vi "UHR-Fleezers Control (host) -Leonardo 04-2018 V1.vi"(0 "Tab Control":T5(tab)=enum."Trap Control (RF)") -> ()   [LabVIEW 2013] (continued)
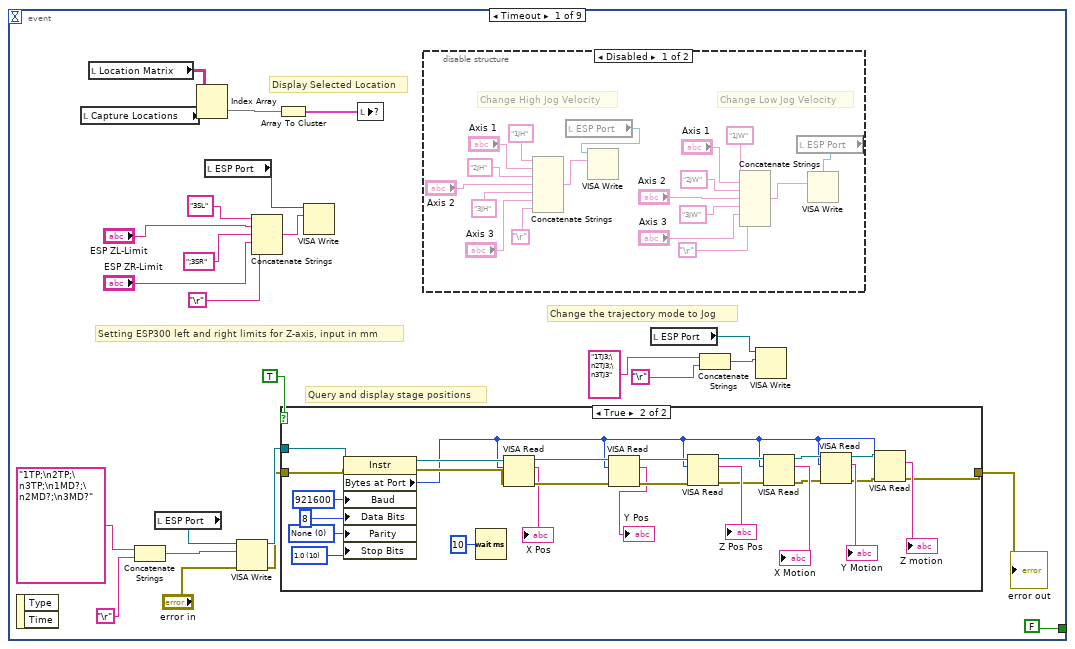
[diagram p2: hidden frame]
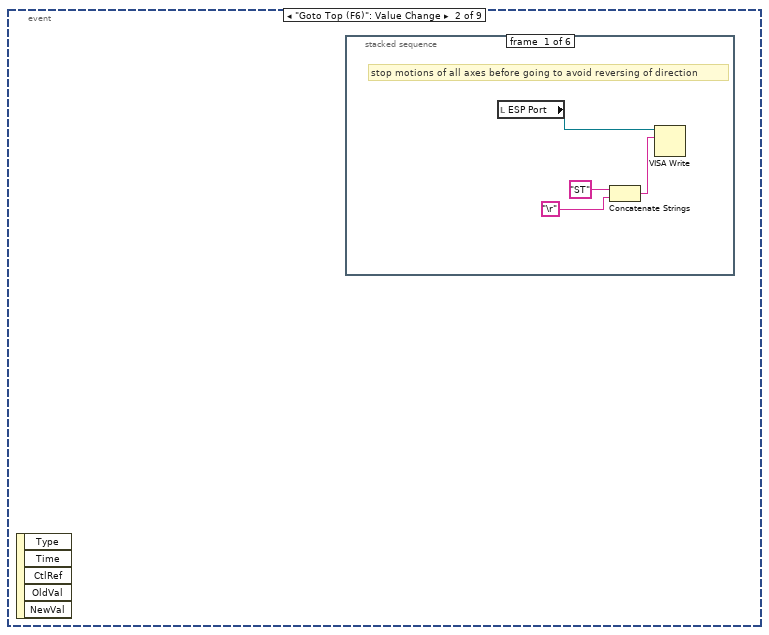
[diagram p5: hidden frame]
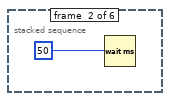
[diagram p6: hidden frame]
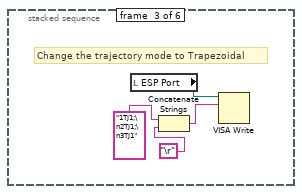
[diagram p7: hidden frame]
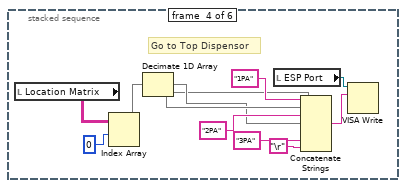
[diagram p8: hidden frame]
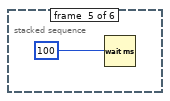
[diagram p9: hidden frame]
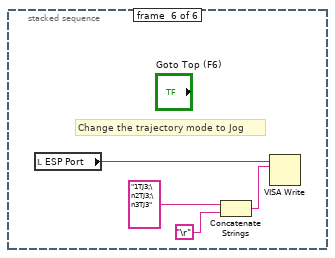
[diagram p10: hidden frame]
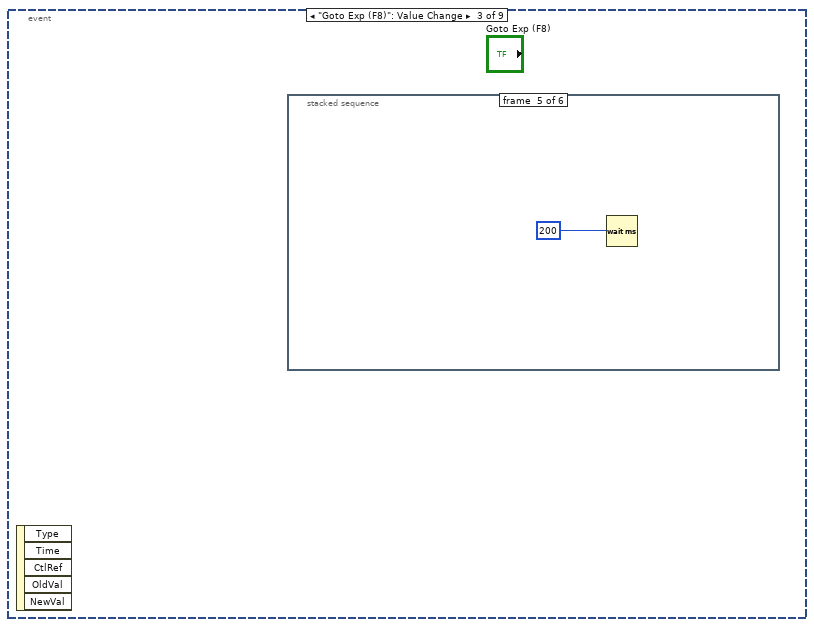
[diagram p11: hidden frame]
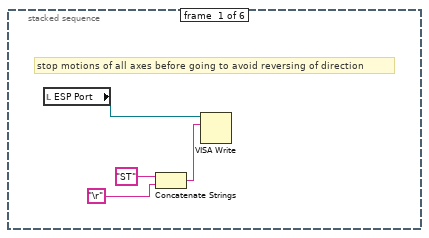
[diagram p12: hidden frame]
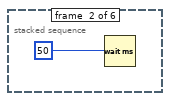
[diagram p13: hidden frame]
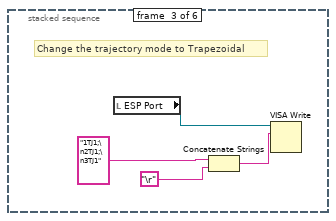
[diagram p14: hidden frame]
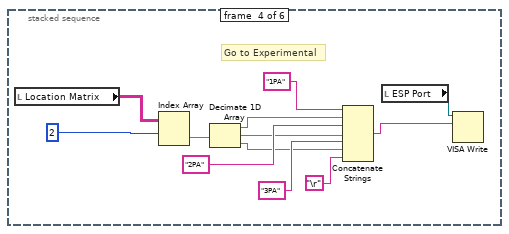
[diagram p15: hidden frame]
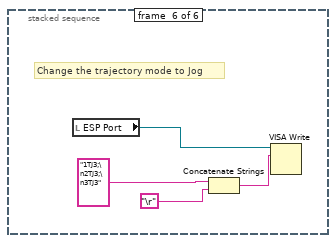
[diagram p16: hidden frame]
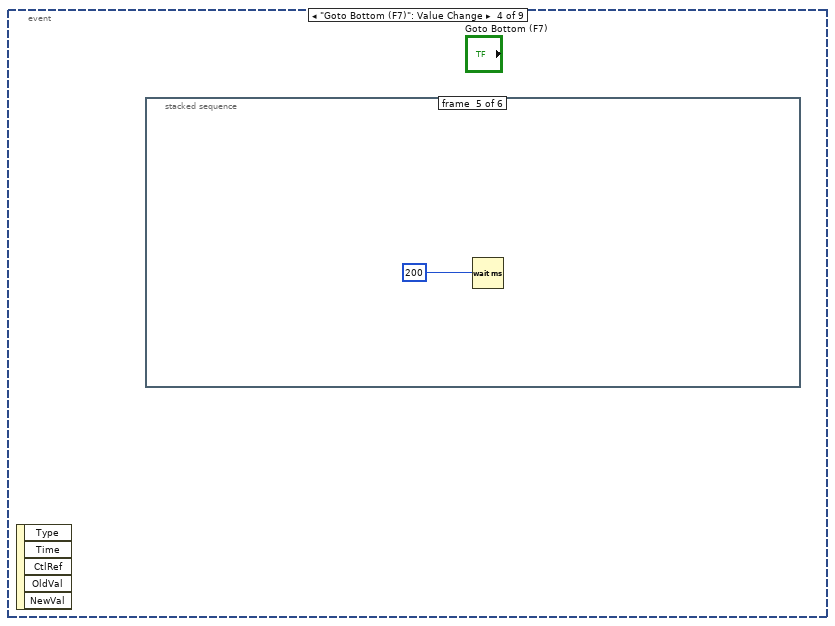
[diagram p17: hidden frame]
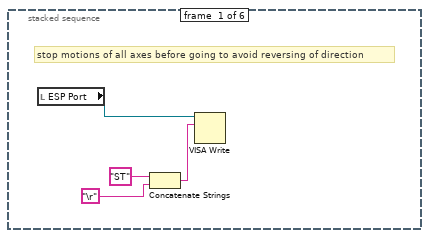
[diagram p18: hidden frame]
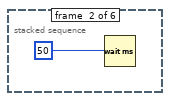
[diagram p19: hidden frame]
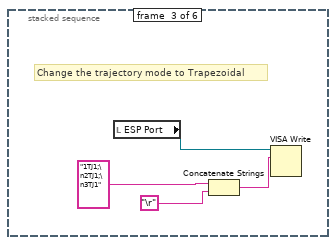
[diagram p20: hidden frame]
                    n2327 = Transpose 2D Array(2D array=w3965) -> (transposed array=w3963:u64[][])
                    n2328 = for {
                      tunnel: w3963 -> [w3968] mode=indexing
                      tunnel: [w3967] -> w3957 mode=indexing
                      tunnel: w3959 -> [w3969]
                      workers-P: _ -> [_]
                      n2329 = call "downsample 1D array - U64.vi"("Ave N"=w3969, "Array In"=w3968) -> ("Array Out"=w3967:u64[])  [unwired: 1 in]
                    }
                    n2330 = Transpose 2D Array(2D array=w3957) -> (transposed array=w3962:u64[][])
                    n2331 = Divide(x=w3960, y=w3959) -> (x/y=w3961:dbl)
                    n2332 = Reshape Array(w3962, w3961) -> (w3958:u64[])
                  }
                }
                n2333 = case shown="True" w3886 {
                  tunnel: w3946 -> [w3978 w3990]
                  tunnel: [w3978 w3982] -> w3942
                  tunnel: "Save ave N" -> [_ w3983]
                  tunnel: w3937 -> [_ w3981]
                  frame False {
                    # "don't downsample data for trap calibration"
                  }
                  frame True {
                    n2334 = Array Size(array=w3990) -> (size(s)=w3984:i32)
                    n2335 = Array Size(array=w3981) -> (size(s)=w3980:i32)
                    n2336 = Divide(x=w3984, y=w3980) -> (x/y=w3988:dbl)
                    n2337 = Reshape Array(w3990, w3988, w3980) -> (w3989:i16[][])
                    n2338 = Transpose 2D Array(2D array=w3989) -> (transposed array=w3987:i16[][])
                    n2339 = for {
                      tunnel: w3987 -> [w3993] mode=indexing
                      tunnel: [w3992] -> w3979 mode=indexing
                      tunnel: w3983 -> [w3991]
                      workers-P: _ -> [_]
                      n2340 = call "downsample 1D array - I16.vi"("Ave N"=w3991, "Array In"=w3993) -> ("Array Out"=w3992:i16[])  [unwired: 1 out]
                    }
                    n2341 = Transpose 2D Array(2D array=w3979) -> (transposed array=w3986:i16[][])
                    n2342 = Divide(x=w3984, y=w3983) -> (x/y=w3985:dbl)
                    n2343 = Reshape Array(w3986, w3985) -> (w3982:i16[])
                  }
                }
                n2344 = Index Array(array=w3908, index=1) -> (element=w3911:waveform(dbl))
                n2345 = Index Array(array=w3908, index=0) -> (element=w3913:waveform(dbl))
                n2346 = Unbundle By Name(w3911) -> ("Y"=w3915:dbl[])
                n2347 = Unbundle By Name(w3913) -> ("Y"=w3923:dbl[])
                n2348 = case "Write trap pos. data" shown="True" w3889 {
                  tunnel: w3888 -> [_ w3971]
                  tunnel: w3884 -> [_ w3970]
                  frame False {
                  }
                  frame True {
                    n2349 = Write to Binary File(file (use dialog)=w3971, data=w3970, 5:FALSE ("prepend array or string size? (T)"), 9:T30."big-endian, network order" ("byte order (0:big-endian, network order)")) -> ()  [unwired: 1 in, 4 out]
                  }
                }
                n2350 = Write to Binary File(file (use dialog)=w3949, data=w3942, 5:FALSE ("prepend array or string size? (T)"), 9:T30."big-endian, network order" ("byte order (0:big-endian, network order)")) -> ()  [unwired: 1 in, 4 out]
                n2351 = feedback #26(w3915) -> (w3917:dbl[])
                n2352 = Build Array (concatenate)(w3917, w3915) -> (w3916:dbl[])
                n2353 = Select(t=w3915, s=w3891, f=w3916) -> (s? t:f=w3901:dbl[])
                n2354 = feedback-in #26(w3901) -> ()
                n2355 = feedback #27(w3923) -> (w3936:dbl[])
                n2356 = Build Array (concatenate)(w3936, w3923) -> (w3935:dbl[])
                n2357 = Select(t=w3923, s=w3891, f=w3935) -> (s? t:f=w3910:dbl[])
                n2358 = feedback-in #27(w3910) -> ()
                n2359 = Divide(x=w3950, y=w3951) -> (x/y=w3953:dbl)
                n2360 = Multiply(x=w3953, y=100.0) -> (x*y=w3952:dbl)
                n2361 = Build Array(w3910, w3901) -> (→"Saved APD":dbl[][])
                n2362 = Array Size(array=w3910) -> (size(s)=w3928:i32)
                n2363 = Unbundle By Name(w3930) -> ("Y"=w3934:dbl[])
                n2364 = Subtract(x=w3928, y="N pts to average") -> (x-y=w3904:i32)
                n2365 = Multiply(x="N pts to average", y=u16 2) -> (x*y=w3905:u16)
                n2366 = Subtract(x=w3928, y=w3905) -> (x-y=w3903:i32)
                n2367 = feedback #28(w3934) -> (w3933:dbl[])
                n2368 = Build Array (concatenate)(w3933, w3934) -> (w3932:dbl[])
                n2369 = Select(t=w3934, s=w3891, f=w3932) -> (s? t:f=w3931:dbl[])
                "Trap Delta Graph" <- w3931
                n2370 = feedback-in #28(w3931) -> ()
                n2371 = Array Subset(array=w3910, index=w3904, length="N pts to average") -> (w3927:dbl[])
                n2372 = Array Subset(array=w3910, index=w3903, length="N pts to average") -> (w3926:dbl[])
                n2373 = Array Subset(array=w3901, index=w3904, length="N pts to average") -> (w3907:dbl[])
                n2374 = Array Subset(array=w3901, index=w3903, length="N pts to average") -> (w3906:dbl[])
                n2375 = call-poly <vilib>:"Mean.vi"("X"=w3927) -> ("mean"=w3925:dbl)  [unwired: 1 out]
                n2376 = call-poly <vilib>:"Mean.vi"("X"=w3907) -> ("mean"=w3900:dbl)  [unwired: 1 out]
                n2377 = call-poly <vilib>:"Mean.vi"("X"=w3926) -> ("mean"=w3924:dbl)  [unwired: 1 out]
                n2378 = call-poly <vilib>:"Mean.vi"("X"=w3906) -> ("mean"=w3899:dbl)  [unwired: 1 out]
                n2379 = Subtract(x=w3900, y=w3899) -> (x-y=w3890:dbl)
                "Delta Fl. 2" <- w3890
                n2380 = Subtract(x=w3925, y=w3924) -> (x-y=w3922:dbl)
                "Delta Fl. 1" <- w3922
                n2381 = Initialize Array(w3922, 1 ("dimension size")) -> (w3919:dbl[])
                n2382 = Initialize Array(w3890, 1 ("dimension size")) -> (w3896:dbl[])
                n2383 = feedback #29(w3919) -> (w3920:dbl[])
                n2384 = Build Array (concatenate)(w3920, w3919) -> (w3918:dbl[])
                n2385 = feedback #30(w3896) -> (w3897:dbl[])
                n2386 = Build Array (concatenate)(w3897, w3896) -> (w3895:dbl[])
                n2387 = Select(t=w3919, s=w3891, f=w3918) -> (s? t:f=w3894:dbl[])
                n2388 = feedback-in #29(w3894) -> ()
                n2389 = Select(t=w3896, s=w3891, f=w3895) -> (s? t:f=w3893:dbl[])
                n2390 = feedback-in #30(w3893) -> ()
                n2391 = Build Array(w3894, w3893) -> (→"Save APD Deriv":dbl[][])
              }
            }
            "Progress" <- w3867
            "Progress 2" <- w3867
          }
        }
      }
    }
    n2392 = Divide(x=w2248, y=w2249) -> (x/y=w2239:ext)
    "Trap 2 amplitude" <- w2239
    n2393 = Bundle By Name(cluster=w2502, "Green FB Ch 0"=w2501, "Green FB Ch 1"=w2500) -> (w2486:T49)
    "Green FB Signals (V)" <- w2486
    n2394 = case shown="True" w2241 {
      tunnel: w2240 -> [_ w2591]
      tunnel: w2239 -> [_ w2590]
      frame False {
      }
      frame True {
        w2592 = 50.0
        n2395 = Greater?(x=w2590, y=w2592) -> (0:w2588:bool)
        n2396 = Greater?(x=w2591, y=w2592) -> (0:w2589:bool)
        n2397 = Or(x=w2589, y=w2588) -> (x .or. y?=w2587:bool)
        n2398 = case shown="True" w2587 {
          frame False {
          }
          frame True {
            n2399 = property on="All FB On/Off" class="Bool (strict)"("Val(Sgnl)"=FALSE) -> ()  [unwired: 2 in, 2 out]
            "Feedback overload" <- TRUE
          }
        }
      }
    }
    n2400 = Unbundle By Name(w2486) -> ("Green FB Ch 2"=→"Green FB Plot":dbl)
    n2401 = local read "wait to reset values"() -> (w2570:bool)
    n2402 = Not(x=w2567) -> (.not. x?=w2571:bool)
    n2403 = And(x=w2571, y=w2570) -> (x .and. y?=w2572:bool)
    n2404 = case "Part of MCL raster scanning: returns to initial positions after scan done" shown="True" w2572 {
      tunnel: w2575 -> [w3416 w3423]
      tunnel: [w3416 w3422] -> w2574
      tunnel: w2569 -> [w3415 w3421]
      tunnel: [w3415 w3420] -> w2568
      frame False {
      }
      frame True {
        w3431 = 10.0 ("y")
        w3430 = 32767.0 ("y")
        # "to return scan values\nafter a synchronous \nAOM scan"
        n2405 = local read "AO2"() -> (w3424:dbl)
        n2406 = local read "AO1"() -> (w3425:dbl)
        n2407 = local write "wait to reset values"(FALSE ("wait to reset values")) -> ()
        n2408 = Multiply(x=w3425, y=w3430) -> (x*y=w3427:dbl)
        n2409 = Multiply(x=w3424, y=w3430) -> (x*y=w3429:dbl)
        n2410 = Divide(x=w3427, y=w3431) -> (x/y=w3426:dbl)
        n2411 = Divide(x=w3429, y=w3431) -> (x/y=w3428:dbl)
        n2412 = To Word Integer(number=w3426) -> (16bit integer=w3432:i16)
        n2413 = To Word Integer(number=w3428) -> (16bit integer=w3433:i16)
        n2414 = local read "Total Counts (ticks)"() -> (w3417:u32)
        n2415 = xnode "Read/Write Control"("FPGA VI Reference In"=w3423, "error in"=w3421, "AO1 (Y)"=w3432, "AO2 (X)"=w3433, "MCL count"=w3417) -> ("FPGA VI Reference Out"=w3422:T20, "error out"=w3420:errorcluster)
        n2416 = local read "Scan Range (V)\n(of steps)"() -> (w3418:dbl)
        n2417 = property on="Scan Range (V)\n(of steps)" class="DigNum (strict)"("Val(Sgnl)"=w3418) -> ()  [unwired: 2 in, 2 out]
      }
    }
    n2418 = node-c288() -> ()  [unwired: 2 out]
  }
  n2419 = node-c288(3 ("Processor")) -> (w107:T25)  [unwired: 3 out]
  n2420 = timed-loop "Oscillate AOD (debugging)" {
    tunnel: w59 -> [w3995]
    tunnel: [w3994] -> w71
    timing: w107 -> [_]
    timing-out: [_] -> w106
    stop <- w3994 stop-if-true
    n2421 = node-c288() -> ()  [unwired: 2 out]
    n2422 = event shown="[0] \"Oscillate Set 2\", \"Fish for Tether\": Value Change" {
      selector: _ -> [_ _ _]
      dyn-events: _ -> [_ _ _]
      timeout: _ -> [_ _ _]
      tunnel: w3995 -> [w4002 _ _]
      tunnel: [FALSE ("Stop All") _ w4270] -> w3994
      event "Oscillate Set 2", "Fish for Tether": Value Change {
        n2423 = event-data() -> ()  [unwired: 6 out]
        n2424 = local read "Oscillate Set 2"() -> (w4001:bool)
        n2425 = Or(x=w4001, y="Fish for Tether") -> (x .or. y?=w3999:bool)
        n2426 = case shown="True" w3999 {
          tunnel: w4002 -> [_ w4005]
          tunnel: "Fish for Tether" -> [_ w4004]
          frame False {
          }
          frame True {
            n2427 = case shown="True" w4004 {
              frame False {
              }
              frame True {
                n2428 = local write "Scan axis 2"(TRUE) -> ()
                n2429 = local write "Tether"(FALSE ("Tether")) -> ()
              }
            }
            n2430 = node-c288("Period") -> (w4007:T25)  [unwired: 3 out]
            n2431 = timed-loop "Oscillate AOD" {
              timing: w4007 -> [_]
              timing-out: [_] -> w4006
              tunnel: w4005 -> [w4017]
              tunnel: w4004 -> [w4016]
              i -> [w4019]
              stop <- w4015 stop-if-true
              n2432 = node-c288() -> (w4018:i64)  [unwired: 1 out]
              n2433 = flat-sequence {
                tunnel: w4019 -> [w4045]
                tunnel: w4018 -> [w4044]
                tunnel: w4017 -> [w4028]
                tunnel: w4016 -> [w4030]
                tunnel: [w4030] -> w4014
                tunnel: [w4029] -> w4013
                tunnel: [w4027] -> w4012
                tunnel: [w4024] -> w4010
                tunnel: w4014 -> [w4081]
                tunnel: w4013 -> [w4079]
                tunnel: w4012 -> [w4078]
                tunnel: [w4077] -> w4011
                tunnel: w4010 -> [w4076]
                tunnel: [w4145] -> w4015
                tunnel: w4011 -> [w4143]
                frame #0 {
                  n2434 = Divide(x=w4044, y=i64 1000) -> (x/y=w4039:dbl)
                  n2435 = Multiply(x=w4039, y=w4045) -> (x*y=w4041:dbl)
                  n2436 = Multiply(x="Osc. freq. (Hz)", y=6.283185307179586) -> (x*y=w4042:dbl)
                  n2437 = Multiply(x=w4042, y=w4041) -> (x*y=w4026:dbl)
                  n2438 = local read "BD 1 Frequency 2 (MHz)"() -> (w4023:dbl)
                  n2439 = local read "BD 1 Frequency 1 (MHz)"() -> (w4020:dbl)
                  n2440 = case shown="True" w4030 {
                    tunnel: w4026 -> [w4051 w4058]
                    tunnel: w4023 -> [_ w4068]
                    tunnel: [w4048 w4052] -> w4031
                    tunnel: [FALSE w4061] -> w4027
                    tunnel: [0.0 w4054] -> w4024
                    tunnel: w4020 -> [_ w4053]
                    frame False {
                      n2441 = Sine(x=w4051) -> (sin(x)=w4049:dbl)
                      n2442 = Multiply(x=w4049, y="Osc. amp. (MHz)") -> (x*y=w4048:dbl)
                    }
                    frame True {
                      n2443 = Cosine(x=w4058) -> (cos(x)=w4071:dbl)
                      n2444 = Subtract(x=w4068, y=w4053) -> (x-y=w4067:dbl)
                      n2445 = Decrement(x=w4071) -> (x-1=w4070:dbl)
                      n2446 = Subtract(x=w4067, y="Closest Delta (MHz)") -> (x-y=w4064:dbl)
                      n2447 = Divide(x=w4070, y=2.0) -> (x/y=w4065:dbl)
                      n2448 = Multiply(x=w4065, y=w4064) -> (x*y=w4052:dbl)
                      n2449 = local read "Vec Mean of T1 T2"() -> (w4060:dbl[])
                      n2450 = Greater?(x=w4060, y="Stop F (pN)") -> (0:w4062:bool[])
                      n2451 = Or Array Elements(Boolean array=w4062) -> (logical OR=w4061:bool)
                      n2452 = Divide(x=w4058, y=6.283185307179586) -> (x/y=w4057:dbl)
                      n2453 = Round Toward +Infinity(x=w4057) -> (ceil(x): smallest int >= x=w4054:dbl)
                      "Attempts" <- w4054
                      n2454 = Greater?(x=w4054, y="Attempt Limit") -> (0:w4056:bool)
                      n2455 = case shown="True" w4056 {
                        frame False {
                        }
                        frame True {
                          n2456 = local write "Fish for Tether"(FALSE ("Fish for Tether")) -> ()
                          n2457 = call <vilib>:"Beep.vi"() -> ()  [unwired: 3 in, 9 out]
                          n2458 = local read "Messages"() -> (w4073:string)
                          n2459 = call "Update messages.vi"("Message to add"="Tether fishing timeout." ("Messages"), "Old message string"=w4073) -> ("New message string"=→"Messages":string)
                        }
                      }
                    }
                  }
                  n2460 = local read "Y RF Frequency Limits (MHz)"() -> (w4032:T16)
                  n2461 = local read "X RF Frequency Limits (MHz)"() -> (w4033:T16)
                  n2462 = local read "BD 1 Frequency 3 (MHz)"() -> (w4038:dbl)
                  n2463 = local read "BD 2 Frequency 2 (MHz)"() -> (w4022:dbl)
                  n2464 = Select(t=w4023, s="Scan axis 2", f=w4022) -> (s? t:f=w4034:dbl)
                  n2465 = Add(x=w4031, y=w4034) -> (x+y=w4029:dbl)
                  n2466 = Select(t=w4029, s="Scan axis 2", f=w4023) -> (s? t:f=w4021:dbl)
                  n2467 = Select(t=w4022, s="Scan axis 2", f=w4029) -> (s? t:f=w4036:dbl)
                  n2468 = local read "BD 2 Frequency 3 (MHz)"() -> (w4037:dbl)
                  n2469 = call "set RF board frequency - interlace.vi"("Board 2 Frequency Limits"=w4032, "Board 1 Frequency Limits"=w4033, "FPGA VI Reference In"=w4028, "Board 2 Frequency 3 (MHz)"=w4037, "Board 1 Frequency 3 (MHz)"=w4038, "Board 2 Frequency 2 (MHz)"=w4022, "Board 2 Frequency 1 (MHz)"=w4036, "Board 1 Frequency 2 (MHz)"=w4021, "Board 1 Frequency 1  (MHz)"=w4020) -> ()  [unwired: 1 in, 2 out]
                }
                frame #1 {
                  n2470 = And(x=w4081, y=w4078) -> (x .and. y?=w4080:bool)
                  n2471 = case "Only if were fishing and now formed tether" shown="True" w4080 {
                    tunnel: w4079 -> [w4083 w4095]
                    tunnel: [w4082 w4094] -> w4077
                    tunnel: w4076 -> [_ w4090]
                    frame False {
                      n2472 = local read "Fish for Tether"() -> (w4082:bool)
                      n2473 = case shown="True" w4082 {
                        tunnel: w4083 -> [_ _]
                        frame False {
                        }
                        frame True {
                        }
                      }
                    }
                    frame True {
                      w4094 = FALSE ("Fish for Tether")
                      n2474 = call <vilib>:"Beep.vi"() -> ()  [unwired: 3 in, 9 out]
                      n2475 = Number To Decimal String(number=w4090, width (-)=i16 1) -> (decimal integer string=w4088:string)
                      n2476 = case shown="\"2\", \"3\", \"4\", \"5\", \"6\"" "Then..." {
                        selector: "Then..." -> [_ w4098]
                        tunnel: w4095 -> [w4097 _]
                        frame "1", Default {
                          # "do nothing"
                          n2477 = property on="BD 1 Frequency 1 (MHz)" class="DigNum (strict)"("Val(Sgnl)"=w4097) -> ()  [unwired: 2 in, 2 out]
                        }
                        frame "2", "3", "4", "5", "6" {
                          n2478 = flat-sequence {
                            tunnel: w4098 -> [w4100]
                            frame #0 {
                              n2479 = property on="Trap Delta (MHz)" class="DigNum (strict)"("Val(Sgnl)"="Move to Delta 1 (MHz)") -> ()  [unwired: 2 in, 2 out]
                            }
                            frame #1 {
                              n2480 = case shown="\"5\", \"6\"" w4100 {
                                selector: w4100 -> [w4103 w4113 _]
                                frame "3", "4" {
                                n2481 = flat-sequence {
                                tunnel: w4103 -> [w4104]
                                tunnel: [w4104] -> w4101
                                tunnel: [w4106] -> w4102
                                tunnel: w4101 -> [w4106]
                                tunnel: w4102 -> [w4110]
                                frame #0 {
                                n2482 = property on="Green Laser ON/Interlacing" class="Bool (strict)"("Val(Sgnl)"=TRUE ("Value (Signaling)")) -> ()  [unwired: 2 in, 2 out]
                                }
                                frame #1 {
                                n2483 = Multiply(x="Wait Before Save (s)", y=u32 1000 ("x")) -> (x*y=w4108:u32)
                                n2484 = Wait (ms)(milliseconds to wait=w4108) -> ()  [unwired: 1 out]
                                }
                                frame #2 {
                                n2485 = property on="Start Saving" class="Bool (strict)"("Value"=TRUE ("Start Saving")) -> ()  [unwired: 2 in, 2 out]
                                n2486 = case shown="Default" w4110 {
                                frame Default {
                                }
                                frame "4" {
                                n2487 = property on="Fl. Triggered..." class="Bool (strict)"("Val(Sgnl)"=TRUE ("Value (Signaling)")) -> ()  [unwired: 2 in, 2 out]
                                }
                                }
                                }
                                }
                                }
                                frame "5", "6" {
                                n2488 = stacked-sequence {
                                tunnel: w4113 -> [_ _ _ _ _ _ _ _ w4130 _ _]
                                frame #0 {
                                n2489 = Replace Array Subset(array=u32[] [0] ("Index Values"), new element="Raster Set Upon Tether", index=0) -> (w4114:u32[])
                                n2490 = property on="Saved AOD Raster Scan Parameter Sets" class="Arr (strict)"("Index Values"=w4114) -> ()  [unwired: 2 in, 2 out]
                                }
                                frame #1 {
                                n2491 = Wait (ms)(milliseconds to wait=u32 500) -> ()  [unwired: 1 out]
                                }
                                frame #2 {
                                n2492 = property on="Load parameters" class="Bool (strict)"("Val(Sgnl)"=TRUE ("Value (Signaling)")) -> ()  [unwired: 2 in, 2 out]
                                }
                                frame #3 {
                                n2493 = Wait (ms)(milliseconds to wait=u32 500) -> ()  [unwired: 1 out]
                                }
                                frame #4 {
                                n2494 = property on="Trap Raster Scan" class="Bool (strict)"("Val(Sgnl)"=TRUE ("Value (Signaling)")) -> ()  [unwired: 2 in, 2 out]
                                }
                                frame #5 {
                                n2495 = Wait (ms)(milliseconds to wait=u32 2000) -> ()  [unwired: 1 out]
                                }
                                frame #6 {
                                n2496 = while {
                                stop <- w4125 stop-if-true
                                n2497 = local read "Raster Scanning..."() -> (w4124:bool)
                                n2498 = local read "Saving..."() -> (w4127:bool)
                                n2499 = Wait (ms)(milliseconds to wait=u32 100) -> ()  [unwired: 1 out]
                                n2500 = Not(x=w4127) -> (.not. x?=w4126:bool)
                                n2501 = Not(x=w4124) -> (.not. x?=w4123:bool)
                                n2502 = And(x=w4126, y=w4123) -> (x .and. y?=w4125:bool)
                                }
                                }
                                frame #7 {
                                n2503 = property on="Trap Delta (MHz)" class="DigNum (strict)"("Val(Sgnl)"="Move to Delta 2 (MHz)") -> ()  [unwired: 2 in, 2 out]
                                }
                                frame #8 {
                                n2504 = local read "Tether"() -> (w4131:bool)
                                n2505 = case shown="True" w4131 {
                                tunnel: w4130 -> [_ w4132]
                                frame False {
                                }
                                frame True {
                                n2506 = flat-sequence {
                                tunnel: w4132 -> [w4134]
                                frame #0 {
                                n2507 = Wait (ms)(milliseconds to wait=u32 500) -> ()  [unwired: 1 out]
                                }
                                frame #1 {
                                n2508 = case shown="\"6\"" w4134 {
                                frame Default {
                                }
                                frame "6" {
                                n2509 = property on="Green Laser ON/Interlacing" class="Bool (strict)"("Val(Sgnl)"=TRUE ("Green Laser ON/Interlacing")) -> ()  [unwired: 2 in, 2 out]
                                }
                                }
                                }
                                frame #2 {
                                n2510 = Wait (ms)(milliseconds to wait=u32 500) -> ()  [unwired: 1 out]
                                }
                                frame #3 {
                                n2511 = local write "Start Saving"("Save at end (5, 6)") -> ()
                                }
                                }
                                }
                                }
                                }
                                frame #9 {
                                n2512 = local read "Bead Sep. Int. Time (s)"() -> (w4140:dbl)
                                n2513 = Multiply(x=w4140, y=1000.0) -> (x*y=w4139:dbl)
                                n2514 = Wait (ms)(milliseconds to wait=w4139) -> ()  [unwired: 1 out]
                                }
                                frame #10 {
                                n2515 = property on="Rescale on Mean" class="Bool (strict)"("Val(Sgnl)"=TRUE ("Value (Signaling)")) -> ()  [unwired: 2 in, 2 out]
                                }
                                }
                                }
                                frame "2", Default {
                                }
                              }
                            }
                          }
                        }
                      }
                      n2516 = Concatenate Strings("Formed tether in ", w4088, " attempt(s)." ("string")) -> (w4085:string)
                      n2517 = local read "Messages"() -> (w4092:string)
                      n2518 = local write "Fish for Tether"(w4094) -> ()
                      n2519 = call "Update messages.vi"("Message to add"=w4085, "Old message string"=w4092) -> ("New message string"=w4091:string)
                      n2520 = local write "Messages"(w4091) -> ()
                      n2521 = Get Date/Time In Seconds() -> (seconds since 1Jan1904=→"Time tether formed":timestamp)
                      "Tether" <- "Tether Alarm?"
                    }
                  }
                }
                frame #2 {
                  n2522 = local read "Oscillate Set 2"() -> (w4144:bool)
                  n2523 = local read "Stop All"() -> (w4146:bool)
                  n2524 = Not Or(1:w4143, 2:w4144) -> (0:w4142:bool)
                  n2525 = Compound Arithmetic op=OR(w4146, w4142) -> (w4145:bool)
                }
              }
              n2526 = node-c288() -> ()  [unwired: 2 out]
            }
            n2527 = node-c288(w4006) -> ()  [unwired: 1 out]
          }
        }
      }
      event "Fl. Triggered...": Value Change {
        n2528 = event-data() -> ()  [unwired: 7 out]
        n2529 = case shown="True" "Fl. Triggered..." {
          frame False {
          }
          frame True {
            n2530 = node-c288() -> (w4158:T25)  [unwired: 4 out]
            n2531 = timed-loop {
              timing: w4158 -> [_]
              timing-out: [_] -> w4157
              tunnel: "Action" -> [w4162]
              shift-right: [w4159] -> _
              shift-left: u8 255 -> [w4161]
              stop <- w4163 stop-if-true
              n2532 = node-c288() -> ()  [unwired: 2 out]
              n2533 = flat-sequence {
                tunnel: w4162 -> [w4175]
                tunnel: w4161 -> [w4172]
                tunnel: [w4171] -> w4160
                tunnel: [w4261] -> w4163
                tunnel: w4160 -> [w4260]
                tunnel: [w4260] -> w4159
                frame #0 {
                  n2534 = local read "Delta Fl. 2"() -> (w4166:dbl)
                  n2535 = local read "Delta Fl. 1"() -> (w4167:dbl)
                  n2536 = Select(t=w4167, s="APD to Watch", f=w4166) -> (s? t:f=w4165:dbl)
                  n2537 = Multiply(x="Fl. Delta Thresh. (kHz)", y=1000.0) -> (x*y=w4174:dbl)
                  n2538 = Greater?(x=w4165, y=w4174) -> (0:w4169:bool)
                  n2539 = Or(x="Force Yank", y=w4169) -> (x .or. y?=w4170:bool)
                  n2540 = case shown="True" w4170 {
                    tunnel: w4175 -> [_ w4185]
                    tunnel: w4172 -> [w4177 w4181]
                    tunnel: [w4177 w4178] -> w4171
                    frame False {
                    }
                    frame True {
                      n2541 = flat-sequence {
                        tunnel: w4182 -> [w4191]
                        tunnel: [w4191] -> w4186
                        tunnel: w4185 -> [w4190]
                        tunnel: [w4190] -> w4184
                        tunnel: [w4189] -> w4183
                        tunnel: w4181 -> [w4188]
                        tunnel: [w4187] -> w4180
                        tunnel: w4186 -> [w4216]
                        tunnel: w4184 -> [w4215]
                        tunnel: w4183 -> [w4214]
                        tunnel: w4180 -> [w4213]
                        tunnel: [w4213] -> w4179
                        tunnel: w4179 -> [w4258]
                        tunnel: [w4258] -> w4178
                        frame #0 {
                          n2542 = call <vilib>:"Beep.vi"() -> ()  [unwired: 3 in, 9 out]
                          n2543 = local write "Waiting"(FALSE ("Waiting")) -> ()
                          n2544 = Increment(x=w4188) -> (x+1=w4187:u8)
                          n2545 = case shown="\"Yank\"" w4190 {
                            tunnel: w4187 -> [_ _ w4197]
                            frame "Image" {
                              n2546 = property on="Confocal Image" class="Bool (strict)"("Val(Sgnl)"=TRUE ("Value (Signaling)")) -> ()  [unwired: 2 in, 2 out]
                            }
                            frame "Alarm", Default {
                            }
                            frame "Yank" {
                              n2547 = flat-sequence {
                                tunnel: w4197 -> [w4200]
                                tunnel: [w4199] -> w4196
                                tunnel: ["N Array El"] -> w4195
                                tunnel: w4196 -> [w4210]
                                tunnel: w4195 -> [w4206]
                                frame #0 {
                                n2548 = Multiply(x="Yank Delay (s)", y=1000.0) -> (x*y=w4203:dbl)
                                n2549 = Quotient & Remainder(x=w4200, y="N Array El") -> (x-y*floor(x/y)=w4199:u8)  [unwired: 1 out]
                                n2550 = Wait (ms)(milliseconds to wait=w4203) -> ()  [unwired: 1 out]
                                }
                                frame #1 {
                                n2551 = Random Number (0-1)() -> (number: 0 to 1=w4207:dbl)
                                n2552 = Multiply(x=w4206, y=w4207) -> (x*y=w4205:dbl)
                                n2553 = Round Toward -Infinity(1:w4205) -> (0:w4204:dbl)
                                n2554 = Select(t=w4204, s="Random Choice", f=w4210) -> (s? t:f=w4208:dbl)
                                n2555 = Index Array(array="Yank to Delta Array (MHz)", index=w4208) -> (element=w4211:dbl)
                                n2556 = property on="Trap Delta (MHz)" class="DigNum (strict)"("Val(Sgnl)"=w4211) -> ()  [unwired: 2 in, 2 out]
                                }
                              }
                            }
                          }
                          n2557 = local read "Time (s)"() -> (w4189:dbl)
                          "Fl. High" <- TRUE ("Yanking")
                        }
                        frame #1 {
                          n2558 = node-c288() -> (w4218:T25)  [unwired: 4 out]
                          n2559 = timed-loop {
                            timing: w4218 -> [_]
                            timing-out: [_] -> w4217
                            tunnel: w4216 -> [w4234]
                            tunnel: w4215 -> [w4232]
                            tunnel: w4214 -> [w4231]
                            stop <- w4233 stop-if-true
                            n2560 = node-c288() -> ()  [unwired: 2 out]
                            n2561 = local read "Fl. Delta Thresh. (kHz)"() -> (w4226:dbl)
                            n2562 = local read "Fl. Triggered..."() -> (w4235:bool)
                            n2563 = local read "Delta Fl. 1"() -> (w4222:dbl)
                            n2564 = local read "Delta Fl. 2"() -> (w4220:dbl)
                            n2565 = local read "Stop All"() -> (w4229:bool)
                            n2566 = local read "APD to Watch"() -> (w4221:bool)
                            n2567 = Select(t=w4222, s=w4221, f=w4220) -> (s? t:f=w4219:dbl)
                            n2568 = Not(x=w4235) -> (.not. x?=w4230:bool)
                            n2569 = Multiply(x=w4226, y=1000.0) -> (x*y=w4225:dbl)
                            n2570 = Negate(x=w4225) -> (-x=w4224:dbl)
                            n2571 = Less?(x=w4219, y=w4224) -> (x < y?=w4228:bool)
                            n2572 = Compound Arithmetic op=OR(w4228, w4229, w4230, "Force Reset") -> (w4233:bool)
                            n2573 = case shown="True" w4233 {
                              tunnel: w4234 -> [_ w4246]
                              tunnel: w4232 -> [_ w4245]
                              tunnel: w4231 -> [_ w4243]
                              frame False {
                              }
                              frame True {
                                n2574 = case shown="\"Yank\"" w4245 {
                                tunnel: w4246 -> [_ w4247]
                                frame "Image", Default {
                                }
                                frame "Yank" {
                                n2575 = flat-sequence {
                                tunnel: [w4252] -> w4248
                                tunnel: w4247 -> [w4252]
                                tunnel: w4248 -> [w4253]
                                frame #0 {
                                n2576 = local read "Yank Delay (s)"() -> (w4251:dbl)
                                n2577 = Multiply(x=w4251, y=1000.0) -> (x*y=w4249:dbl)
                                n2578 = Wait (ms)(milliseconds to wait=w4249) -> ()  [unwired: 1 out]
                                }
                                frame #1 {
                                n2579 = property on="Trap Delta (MHz)" class="DigNum (strict)"("Val(Sgnl)"=w4253) -> ()  [unwired: 2 in, 2 out]
                                }
                                }
                                }
                                }
                                n2580 = local read "Time (s)"() -> (w4244:dbl)
                                n2581 = Subtract(x=w4244, y=w4243) -> (x-y=w4240:dbl)
                                "Duration (s)" <- w4240
                                n2582 = Number To Decimal String(number=w4240, width (-)=i16 0) -> (decimal integer string=w4238:string)
                                n2583 = Concatenate Strings(w4238, " s fluorescence event." ("string")) -> (w4236:string)
                                n2584 = local read "Messages"() -> (w4242:string)
                                n2585 = call "Update messages.vi"("Message to add"=w4236, "Old message string"=w4242) -> ("New message string"=w4241:string)
                                n2586 = call <vilib>:"Beep.vi"() -> ()  [unwired: 3 in, 9 out]
                                n2587 = local write "Messages"(w4241) -> ()
                              }
                            }
                            n2588 = node-c288() -> ()  [unwired: 2 out]
                          }
                          n2589 = node-c288(w4217) -> ()  [unwired: 1 out]
                        }
                        frame #2 {
                          n2590 = local write "Fl. High"(FALSE ("Yanking")) -> ()
                        }
                      }
                      n2591 = local read "Trap Delta (MHz)"() -> (w4182:dbl)
                    }
                  }
                }
                frame #1 {
                  n2592 = local read "Stop All"() -> (w4264:bool)
                  n2593 = local read "Fl. Triggered..."() -> (w4262:bool)
                  n2594 = Not(x=w4262) -> (.not. x?=w4263:bool)
                  n2595 = Or(x=w4263, y=w4264) -> (x .or. y?=w4261:bool)
                  n2596 = Not(x=w4261) -> (.not. x?=→"Waiting":bool)
                }
              }
              n2597 = node-c288() -> ()  [unwired: 2 out]
            }
            n2598 = node-c288(w4157) -> ()  [unwired: 1 out]
          }
        }
      }
      event "Stop All": Value Change {
        n2599 = event-data() -> ()  [unwired: 7 out]
        n2600 = local read "Stop All"() -> (w4270:bool)
      }
    }
    n2601 = node-c288() -> ()  [unwired: 2 out]
  }
  n2602 = node-c288(w106) -> ()  [unwired: 1 out]
  n2603 = node-c288(w193) -> ()  [unwired: 1 out]
  n2604 = flat-sequence {
    tunnel: w68 -> [w4275]
    tunnel: [w4274] -> w74
    tunnel: [w4271] -> w73
    tunnel: w72 -> [_]
    tunnel: w71 -> [_]
    tunnel: w70 -> [_]
    tunnel: w69 -> [_]
    tunnel: w67 -> [w4272]
    tunnel: w74 -> [w4278]
    tunnel: w73 -> [w4277]
    frame #0 {
      w4273 = FALSE ("APD to FIFO")
      n2605 = xnode "Read/Write Control"("FPGA VI Reference In"=w4275, "error in"=w4272, "APD to FIFO"=w4273, "AI to FIFO"=w4273) -> ("FPGA VI Reference Out"=w4274:T20, "error out"=w4271:errorcluster)
    }
    frame #1 {
      n2606 = xnode "Invoke Method"("FPGA VI Reference In"=w4278, "error in"=w4277) -> ("FPGA VI Reference Out"=w4276:T20)  [unwired: 1 out]
      n2607 = xnode "Close FPGA VI Reference"("FPGA VI Reference In"=w4276) -> ()  [unwired: 1 in, 1 out]
    }
  }
